vi "Newton_New x0.vi"(6 "new x0":dbl, 8 "x0 in":dbl, 9 "new P(x0)":dbl, 10 "noise in":i32, 11 "|P(x0)| in":dbl) -> (1 "x0 out":dbl, 2 "noise out":i32, 3 "|P(x0)| out":dbl)   [LabVIEW 2017, in "NI_AALPro.lvlib"]
uses:
  NI_AALPro.lvlib
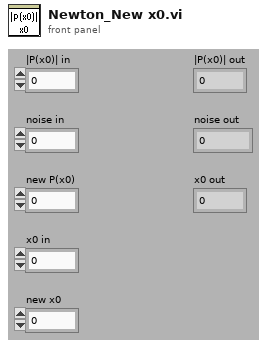
[diagram p1: front panel]
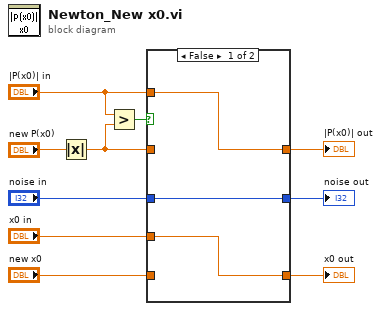
[diagram p0: block diagram]
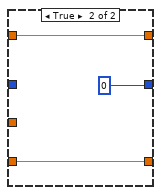
[diagram p2: hidden frame]
diagram:
  n1 = Absolute Value(x="new P(x0)") -> (abs(x)=w10:dbl)
  n2 = Greater?(x="|P(x0)| in", y=w10) -> (0:w4:bool)
  n3 = case shown="False" w4 {
    tunnel: "|P(x0)| in" -> [w13 _]
    tunnel: w10 -> [_ w16]
    tunnel: "new x0" -> [_ w15]
    tunnel: "x0 in" -> [w12 _]
    tunnel: "noise in" -> [w11 _]
    tunnel: [w13 w16] -> w2
    tunnel: [w12 w15] -> w3
    tunnel: [w11 0] -> w1
    frame False {
    }
    frame True {
    }
  }
  "x0 out" <- w3
  "|P(x0)| out" <- w2
  "noise out" <- w1
